vi "Read Font Size.vi"(8 "error in (no error)":errorcluster, 11 "Code String in":refnum<class "Code String.lvclass">) -> (0 "error out":errorcluster, 2 "Font Size":u32, 3 "Code String out":refnum<class "Code String.lvclass">)   [LabVIEW 2016, in "Code String.lvclass"]
doc: "Reads the <b>Font Size</b> from the Code String.\n--------------------\nCopyright (c) 2019 Analog Devices, Inc. All rights reserved.\n\nRedistribution and use in source and binary forms, with or without modification,\nare permitted provided that the following conditions are met:\n - Redistributions of source code must retain the above copyright notice, this\n list of conditions and the following disclaimer.\n - Redistributions in binary form must reproduce the above copyright notice,\n this list of conditions and the following disclaimer in the documentation\n and/or other materials provided with the distribution.\n - Modified versions of the software must be conspicuously marked as such.\n - This software is licensed solely and exclusively for use with\n processors/products manufactured by or for Analog Devices, Inc.\n - This software may not be combined or merged with other code in any manner\n that would cause the software to become subject to terms and conditions\n which differ from those listed here.\n - Neither the name of Analog Devices, Inc. nor the names of its contributors\n may be used to endorse or promote products derived from this software\n without specific prior written permission.\n - The use of this software may or may not infringe the patent rights of one or\n more patent holders. This license does not release you from the requirement\n that you obtain separate licenses from these patent holders to use this\n software.\n\nTHIS SOFTWARE IS PROVIDED BY ANALOG DEVICES, INC. AND CONTRIBUTORS \"AS IS\" AND\nANY EXPRESS OR IMPLIED WARRANTIES, INCLUDING, BUT NOT LIMITED TO,\nNON-INFRINGEMENT, TITLE, MERCHANTABILITY AND FITNESS FOR A PARTICULAR PURPOSE\nARE DISCLAIMED. IN NO EVENT SHALL ANALOG DEVICES, INC. OR CONTRIBUTORS BE LIABLE\nFOR ANY DIRECT, INDIRECT, INCIDENTAL, SPECIAL, EXEMPLARY, PUNITIVE OR\nCONSEQUENTIAL DAMAGES (INCLUDING, BUT NOT LIMITED TO, DAMAGES ARISING OUT OF\nCLAIMS OF INTELLECTUAL PROPERTY RIGHTS INFRINGEMENT; PROCUREMENT OF SUBSTITUTE\nGOODS OR SERVICES; LOSS OF USE, DATA, OR PROFITS; OR BUSINESS INTERRUPTION)\nHOWEVER CAUSED AND ON ANY THEORY OF LIABILITY, WHETHER IN CONTRACT, STRICT\nLIABILITY, OR TORT (INCLUDING NEGLIGENCE OR OTHERWISE) ARISING IN ANY WAY OUT OF\nTHE USE OF THIS SOFTWARE, EVEN IF ADVISED OF THE POSSIBILITY OF SUCH DAMAGE.\n\n2019-01-10-7CBSD SLA"
uses:
  Code String.lvclass
  Font Global.vi
panel:
  # "Copyright (c) 2019 Analog Devices, Inc.  All rights reserved.\n\nRedistribution and use in source and binary forms, with or without modification,\nare permitted provided that the following conditions are met:\n  - Redistributions of source code must retain the above copyright notice, this\n    list of conditions and the following disclaimer.\n  - Redistributions in binary form must reproduce the above copyright notice,\n    this list of conditions and the following disclaimer in the documentation\n    and/or other materials provided with the distribution.\n  - Modified versions of the software must be conspicuously marked as such.\n  - This software is licensed solely and exclusively for use with\n    processors/products manufactured by or for Analog Devices, Inc.\n  - This software may not be combined or merged with other code in any manner\n    that would cause the software to become subject to terms and conditions\n    which differ from those listed here.\n  - Neither the name of Analog Devices, Inc. nor the names of its contributors\n    may be used to endorse or promote products derived from this software\n    without specific prior written permission.\n  - The use of this software may or may not infringe the patent rights of one or\n    more patent holders.  This license does not release you from the requirement\n    that you obtain separate licenses from these patent holders to use this\n    software.\n\nTHIS SOFTWARE IS PROVIDED BY ANALOG DEVICES, INC. AND CONTRIBUTORS \"AS IS\" AND\nANY EXPRESS OR IMPLIED WARRANTIES, INCLUDING, BUT NOT LIMITED TO,\nNON-INFRINGEMENT, TITLE, MERCHANTABILITY AND FITNESS FOR A PARTICULAR PURPOSE\nARE DISCLAIMED. IN NO EVENT SHALL ANALOG DEVICES, INC. OR CONTRIBUTORS BE LIABLE\nFOR ANY DIRECT, INDIRECT, INCIDENTAL, SPECIAL, EXEMPLARY, PUNITIVE OR\nCONSEQUENTIAL DAMAGES (INCLUDING, BUT NOT LIMITED TO, DAMAGES ARISING OUT OF\nCLAIMS OF INTELLECTUAL PROPERTY RIGHTS INFRINGEMENT; PROCUREMENT OF SUBSTITUTE\nGOODS OR SERVICES; LOSS OF USE, DATA, OR PROFITS; OR BUSINESS INTERRUPTION)\nHOWEVER CAUSED AND ON ANY THEORY OF LIABILITY, WHETHER IN CONTRACT, STRICT\nLIABILITY, OR TORT (INCLUDING NEGLIGENCE OR OTHERWISE) ARISING IN ANY WAY OUT OF\nTHE USE OF THIS SOFTWARE, EVEN IF ADVISED OF THE POSSIBILITY OF SUCH DAMAGE.\n\n2019-01-10-7CBSD SLA"
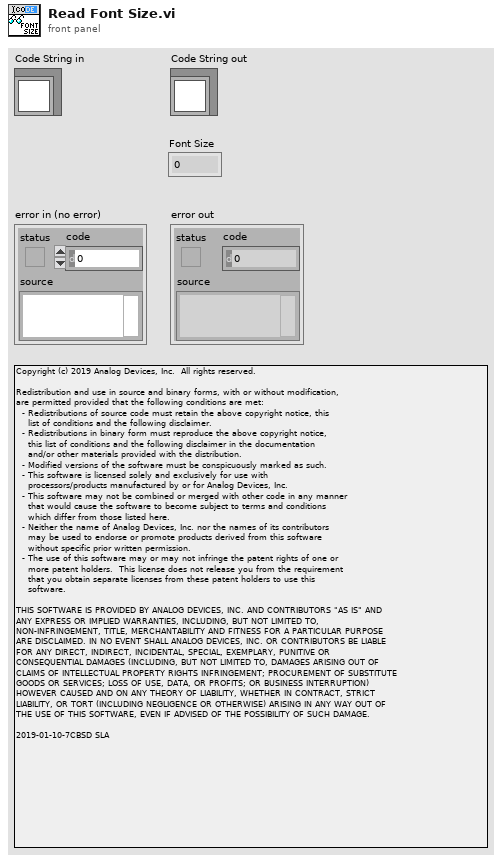
[diagram p1: front panel]
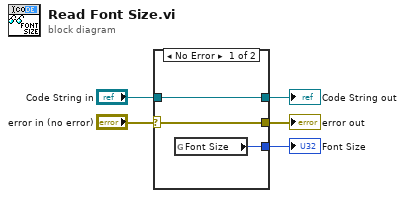
[diagram p0: block diagram]
diagram:
  n1 = case shown="No Error" "error in (no error)" {
    selector: "error in (no error)" -> [w7 w10]
    tunnel: [w7 w10] -> w4
    tunnel: [w8 w9] -> w2
    tunnel: "Code String in" -> [w8 w9]
    tunnel: [w6 _] -> w1
    frame No Error {
      n2 = global read "Font Global.vi" "Font Size"() -> (w6:u32)
    }
    frame Error {
    }
  }
  "error out" <- w4
  "Code String out" <- w2
  "Font Size" <- w1
